vi "Initiate.vi"(8 "error in (no error)":errorcluster, 11 "VISA resource name":refnum<visa-resource-name>) -> (0 "error out":errorcluster, 3 "VISA resource name out":refnum<visa-resource-name>)   [LabVIEW 2018, in "Suita SPAW7000.lvlib"]
doc: "Initiates a measurement based on the preset configuration. The measurement type must be configured before calling this function. This is accomplished by calling the <b>Configure Measurement</b> VI. After the <b>Initiate</b> VI is called, the Power Meter leaves the Idle state and waits for a trigger.\n\n<B>Note:</B> Use this VI only with other low-level VIs. The high-level VIs automatically incorporate this functionality. This VI does not check the instrument status."
uses:
  <instrlib>/Suita SPAW7000/Suita SPAW7000.lvlib
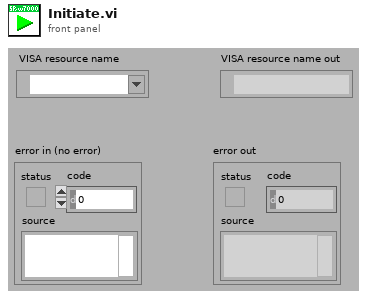
[diagram p1: front panel]
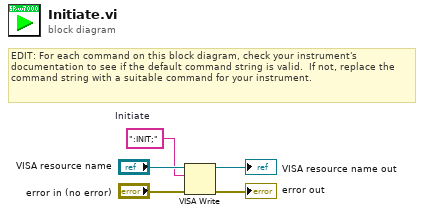
[diagram p0: block diagram]
diagram:
  w3 = ":INIT;"  # Initiate
  # "EDIT: For each command on this block diagram, check your instrument's  documentation to see if the default command string is valid.  If not, replace the command string with a suitable command for your instrument."
  n1 = VISA Write(VISA resource name="VISA resource name", write buffer=w3, error in (no error)="error in (no error)") -> (VISA resource name out=→"VISA resource name out":refnum<visa-resource-name>, error out=→"error out":errorcluster)  [unwired: 1 out]
